vi "MI-Run.vi"() -> ()   [LabVIEW 2010]
panel:
  in  "iowkit.dll path":path=path "C:/Users/sira01/Documents/AirBathCTL_2/iowkit api/x64/iowkit.dll"
  in  "Vor-Temperatur":dbl[unit]=296.15 min=283.15 max=313.15 step=1.0
  out "Code":u16=563 format="%03x"
  out "aktuelle Temperatur":dbl[unit]=23.0
  in  "Startzeit":enum16{"Sofort", "Später"}(ring)
  in  "Start":timestamp=timestamp(3549967200.8880715 s since 1904-01-01) format="%<%H:%M:%S\n%x>T"
  out "Uhrzeit":timestamp[](array[timestamp])=[timestamp(3549974578.9889793 s since 1904-01-01), timestamp(3549990778.9889793 s since 1904-01-01), timestamp(3550006978.9889793 s since 1904-01-01), timestamp(3550023178.9889793 s since 1904-01-01), timestamp(3550066378.9889793 s since 1904-01-01), timestamp(3550082578.9889793 s since 1904-01-01), timestamp(3550098778.9889793 s since 1904-01-01), timestamp(3550114978.9889793 s since 1904-01-01)] caption="Daten" format="%<%H:%M:%S\n%x>T"
  in  "Cluster":T1={"Temperatur"=[296.15, 298.15, 294.15, 296.15, 300.15, 292.15, 296.15], "Dauer"=[16200.0, 16200.0, 16200.0, 43200.0, 16200.0, 16200.0, 16200.0]} {"Dauer" format="%#.3f"; "Temperatur" format="%#.3f"}
  in  "Polynom-Grad":i32=3 min=1 max=8 step=1
  out "err out":errorcluster caption="error"
  out "Raw Data and Fitted Curve":cluster{dbl[], "Best Exponential Fit":dbl[]}[](graph)=[{[19.08, 21.2, 22.22, 23.25, 24.145, 25.28, 27.25], "Best Exponential Fit"=[72.68, 62.91, 58.35, 53.99, 49.81, 45.81, 38.29]}, {[19.08, 21.2, 22.22, 23.25, 24.145, 25.28, 27.25], "Best Exponential Fit"=[72.69152397945143, 62.887051630235376, 58.334339275352725, 53.87656342649992, 50.13486284759349, 45.59096817055149, 38.32469066404728]}] caption="Poti-Position / %"
  in  "Mode":T2(ring)
  # "Temperatur            Dauer"
  # "°C"
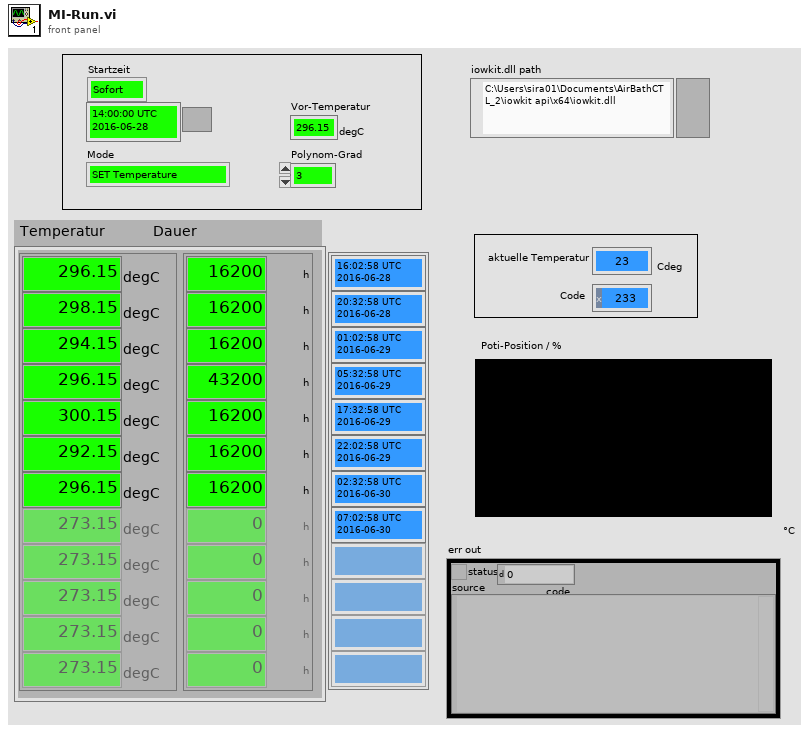
[diagram p1: front panel]
types:
  T1 = cluster{"Temperatur":dbl[unit][], "Dauer":dbl[unit][]}
  T2 = enum16{"SET Temperature", "START Temperature-Array", "CLEAR Array"}
  T3 = enum16{"Temperaturfit", "aus Datei lesen", "in Datei Schreiben"}
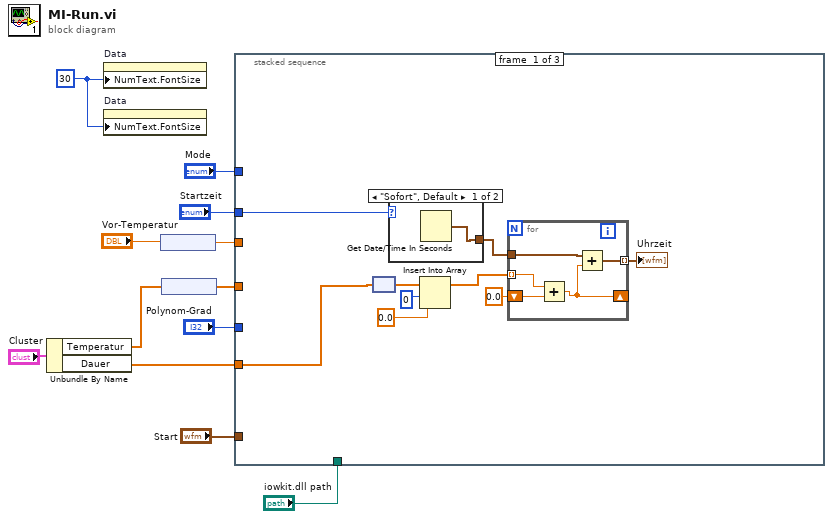
[diagram p0: block diagram]
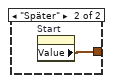
[diagram p2: hidden frame]
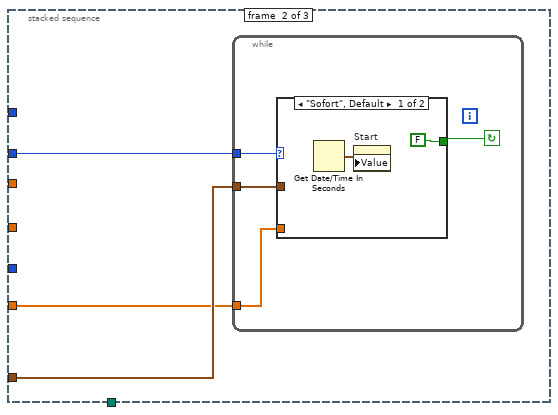
[diagram p3: hidden frame]
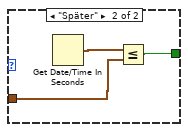
[diagram p4: hidden frame]
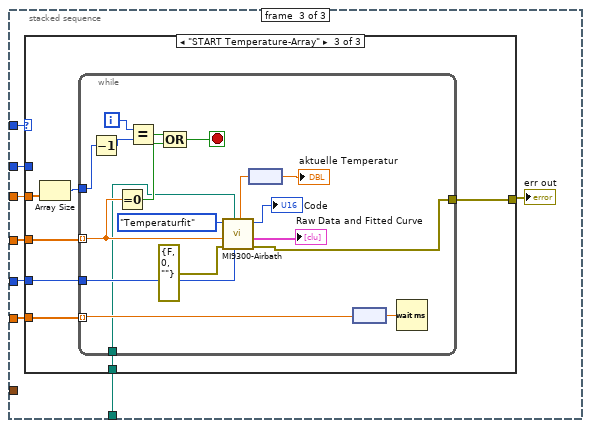
[diagram p5: hidden frame]
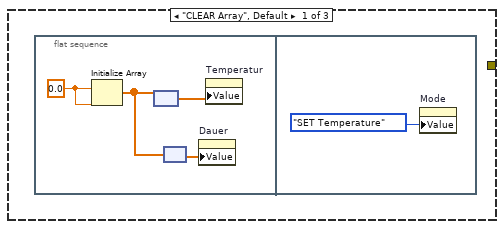
[diagram p6: hidden frame]
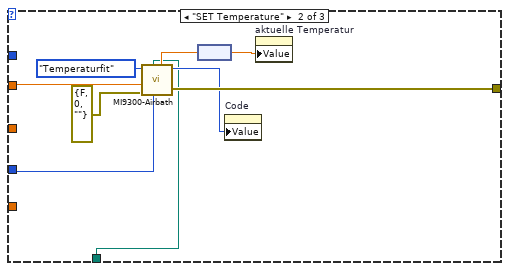
[diagram p7: hidden frame]
diagram:
  w8 = u32 30 ("Beschriftung.Schriftart:Größe")
  n1 = Unbundle By Name("Cluster") -> ("Temperatur"=w10:dbl[unit][], "Dauer"=w3:dbl[unit][])
  n2 = property on="Data" class="DigNum (strict)"("NumText.FontSize"=w8) -> ()  [unwired: 2 in, 2 out]
  n3 = property on="Data" class="DigNum (strict)"("NumText.FontSize"=w8) -> ()  [unwired: 2 in, 2 out]
  n4 = node("Vor-Temperatur") -> (w5:dbl)
  n5 = node(w10) -> (w9:dbl[])
  n6 = stacked-sequence {
    tunnel: "Mode" -> [_ _ w48]
    tunnel: w3 -> [w13 w29 w47]
    tunnel: w9 -> [_ _ w46]
    tunnel: "Polynom-Grad" -> [_ _ w44]
    tunnel: w5 -> [_ _ w43]
    tunnel: "Startzeit" -> [w14 w30 w42]
    tunnel: "Start" -> [_ w31 _]
    tunnel: "iowkit.dll path" -> [_ _ w41]
    frame #0 {
      n7 = node(w13) -> (w19:dbl[])
      n8 = case shown="\"Sofort\", Default" w14 {
        tunnel: [w22 w23] -> w21
        frame "Sofort", Default {
          n9 = Get Date/Time In Seconds() -> (seconds since 1Jan1904=w22:timestamp)
        }
        frame "Später" {
          n10 = property on="Start" class="AbsTime (strict)"() -> ("Value"=w23:timestamp)  [unwired: 2 in, 2 out]
        }
      }
      n11 = Insert Into Array(array=w19, index=0 ("Index"), new element=0.0 ("Neues Element/Teil-Array")) -> (w20:dbl[])
      n12 = for {
        tunnel: w20 -> [w26] mode=indexing
        tunnel: [w28] -> w15 mode=indexing
        shift-right: [w25] -> _
        shift-left: 0.0 -> [w27]
        tunnel: w21 -> [w24]
        n13 = Add(x=w26, y=w27) -> (x+y=w25:dbl)
        n14 = Add(x=w24, y=w25) -> (x+y=w28:timestamp)
      }
      "Uhrzeit" <- w15
    }
    frame #1 {
      n15 = while {
        tunnel: w30 -> [w34]
        tunnel: w29 -> [w33]
        tunnel: w31 -> [w32]
        stop <- w35 continue-if-true
        n16 = case shown="\"Sofort\", Default" w34 {
          tunnel: [FALSE w39] -> w35
          tunnel: w33 -> [_ _]
          tunnel: w32 -> [_ w38]
          frame "Sofort", Default {
            n17 = Get Date/Time In Seconds() -> (seconds since 1Jan1904=w36:timestamp)
            n18 = property on="Start" class="AbsTime (strict)"("Value"=w36) -> ()  [unwired: 2 in, 2 out]
          }
          frame "Später" {
            n19 = Get Date/Time In Seconds() -> (seconds since 1Jan1904=w40:timestamp)
            n20 = Less Or Equal?(x=w40, y=w38) -> (x <= y?=w39:bool)
          }
        }
      }
    }
    frame #2 {
      n21 = case shown="\"START Temperature-Array\"" w48 {
        tunnel: w47 -> [_ _ w67]
        tunnel: w46 -> [_ _ w68]
        tunnel: w43 -> [_ w62 _]
        tunnel: [_ w61 w66] -> w45
        tunnel: w44 -> [_ w60 w65]
        tunnel: w42 -> [_ _ _]
        tunnel: w41 -> [_ w54 w63]
        frame "CLEAR Array", Default {
          n22 = flat-sequence {
            frame #0 {
              w51 = 0.0 ("Element")
              n23 = Initialize Array(w51, w51) -> (w49:dbl[])
              n24 = node(w49) -> (w50:dbl[unit][])
              n25 = node(w49) -> (w52:dbl[unit][])
              n26 = property on="Dauer" class="Arr (strict)"("Value"=w52) -> ()  [unwired: 2 in, 2 out]
              n27 = property on="Temperatur" class="Arr (strict)"("Value"=w50) -> ()  [unwired: 2 in, 2 out]
            }
            frame #1 {
              n28 = property on="Mode" class="Enum (strict)"("Value"=T2."SET Temperature" ("Mode")) -> ()  [unwired: 2 in, 2 out]
            }
          }
        }
        frame "SET Temperature" {
          n29 = call "MI9300-Airbath.vi"("Polynom-Grad"=w60, "iowkit.dll path"=w54, "err in"=errorcluster {"status"=FALSE, "code"=0, "source"=""} ("error in (no error)"), "Temperatur"=w62, "Option"=T3."Temperaturfit") -> ("err out"=w61:errorcluster, "Code"=w58:u16, "Temperatur_out"=w57:dbl)  [unwired: 2 in, 2 out]
          n30 = node(w57) -> (w56:dbl[unit])
          n31 = property on="Code" class="DigNum (strict)"("Value"=w58) -> ()  [unwired: 2 in, 2 out]
          n32 = property on="aktuelle Temperatur" class="DigNum (strict)"("Value"=w56) -> ()  [unwired: 2 in, 2 out]
        }
        frame "START Temperature-Array" {
          n33 = Array Size(array=w68) -> (size(s)=w64:i32)
          n34 = while {
            tunnel: w68 -> [w82] mode=indexing
            tunnel: w67 -> [w73] mode=indexing
            tunnel: [w75] -> w66
            tunnel: w65 -> [w74]
            tunnel: w64 -> [w71]
            tunnel: w63 -> [w69]
            i -> [w81]
            stop <- w79 stop-if-true
            n35 = Decrement(x=w71) -> (x-1=w84:i32)
            n36 = Equal To 0?(x=w82) -> (x = 0?=w80:bool)
            n37 = Equal?(x=w81, y=w84) -> (x = y?=w83:bool)
            n38 = Compound Arithmetic op=OR(w83, w80) -> (w79:bool)
            n39 = call "MI9300-Airbath.vi"("Polynom-Grad"=w74, "iowkit.dll path"=w69, "err in"=errorcluster {"status"=FALSE, "code"=0, "source"=""} ("error in (no error)"), "Temperatur"=w82, "Option"=T3."Temperaturfit") -> ("err out"=w75:errorcluster, "Raw Data and Fitted Curve"=→"Raw Data and Fitted Curve":cluster{dbl[], "Best Exponential Fit":dbl[]}[], "Code"=→"Code":u16, "Temperatur_out"=w78:dbl)  [unwired: 2 in, 1 out]
            n40 = node(w78) -> (→"aktuelle Temperatur":dbl[unit])
            n41 = node(w73) -> (w72:dbl)
            n42 = Wait (ms)(milliseconds to wait=w72) -> ()  [unwired: 1 out]
          }
        }
      }
      "err out" <- w45
    }
  }
